vi "nanocal -- nuclear schottky fit V7.vi"() -> ()   [LabVIEW 2021] (continued)
\"B\" -> 0.000000000000   ,  \"θ\" -> 0.000000000000   ,  \"Reoff\" -> -959183.673469387924   ,  \"Imoff\" -> 0.000000000000   ,  \"στ1\" -> 0.000056019641   ,  \"στS\" -> 0.002791706038   ,  \"στN\" -> 0.000000650322    |>   , \r\"IDS0417_220525_RAW_cal__sam_\" ->   <|    \"ζ\" -> 0.020422056832   ,  \"τ1\" -> 0.006457484957   ,  \"τS\" -> 0.019722165301   ,  \"τN\" -> 0.000729413719   ,  \"τC\" -> 0.001622930071   ,  \"κ0\" -> 0.000000005380   ,  \"mm1\" -> 0.000030097695   ,  \"mm2\" -> 0.006162713408   ,  \"mm3\" -> 0.022756846254   ,  \"T\" -> 0.830000000000   ,  \"B\" -> 0.000000000000   ,  \"θ\" -> 0.000000000000   ,  \"Reoff\" -> -2081632.653061224150   ,  \"Imoff\" -> 0.000000000000   ,  \"στ1\" -> 0.000977899540   ,  \"στS\" -> 0.002370947727   ,  \"στN\" -> 0.000160479256    |>   , \r\"IDS0418_220525_RAW_cal__ref_\" ->   <|    \"ζ\" -> 0.101578237405   ,  \"τ1\" -> 0.000131000000   ,  \"τS\" -> 0.019496503151   ,  \"τN\" -> 0.000001000000   ,  \"τC\" -> 0.002824938622   ,  \"κ0\" -> 0.000000006490   ,  \"mm1\" -> 0.000130992305   ,  \"mm2\" -> 0.000232437503   ,  \"mm3\" -> 0.024070533970   ,  \"T\" -> 1.120000000000   ,  \"B\" -> 0.000000000000   ,  \"θ\" -> 0.000000000000   ,  \"Reoff\" -> -9469387.755102038390   ,  \"Imoff\" -> 0.000000000000   ,  \"στ1\" -> 0.000013096925   ,  \"στS\" -> 0.001629413974   ,  \"στN\" -> 0.000000279483    |>   , \r\"IDS0418_220525_RAW_cal__sam_\" ->   <|    \"ζ\" -> 0.010833914814   ,  \"τ1\" -> 0.006105280968   ,  \"τS\" -> 0.027771405990   ,  \"τN\" -> 0.000655710517   ,  \"τC\" -> 0.001898693697   ,  \"κ0\" -> 0.000000007420   ,  \"mm1\" -> 0.000019072683   ,  \"mm2\" -> 0.005941306089   ,  \"mm3\" -> 0.030778689359   ,  \"T\" -> 1.120000000000   ,  \"B\" -> 0.000000000000   ,  \"θ\" -> 0.000000000000   ,  \"Reoff\" -> -608163.265306122367   ,  \"Imoff\" -> 0.000000000000   ,  \"στ1\" -> 0.001326459237   ,  \"στS\" -> 0.003728359065   ,  \"στN\" -> 0.000181682896    |>   , \r\"IDS0419_220525_RAW_cal__ref_\" ->   <|    \"ζ\" -> 0.054328127598   ,  \"τ1\" -> 0.000131000000   ,  \"τS\" -> 0.041800630964   ,  \"τN\" -> 0.000001000000   ,  \"τC\" -> 0.008136787294   ,  \"κ0\" -> 0.000000011908   ,  \"mm1\" -> 0.000130996584   ,  \"mm2\" -> 0.000356366999   ,  \"mm3\" -> 0.051853059016   ,  \"T\" -> 1.900000000000   ,  \"B\" -> 0.000000000000   ,  \"θ\" -> 0.000000000000   ,  \"Reoff\" -> -2412244.897959183900   ,  \"Imoff\" -> 0.000000000000   ,  \"στ1\" -> 0.000075606348   ,  \"στS\" -> 0.006052354245   ,  \"στN\" -> 0.000000670558    |>   , \r\"IDS0419_220525_RAW_cal__sam_\" ->   <|    \"ζ\" -> 0.011595776290   ,  \"τ1\" -> 0.006117918264   ,  \"τS\" -> 0.061916055974   ,  \"τN\" -> 0.000669101537   ,  \"τC\" -> 0.002022450323   ,  \"κ0\" -> 0.000000012950   ,  \"mm1\" -> 0.000022465670   ,  \"mm2\" -> 0.006048051710   ,  \"mm3\" -> 0.065380732203   ,  \"T\" -> 1.900000000000   ,  \"B\" -> 0.000000000000   ,  \"θ\" -> 0.000000000000   ,  \"Reoff\" -> -608163.265306122367   ,  \"Imoff\" -> 0.000000000000   ,  \"στ1\" -> 0.001547930555   ,  \"στS\" -> 0.007827805463   ,  \"στN\" -> 0.000227173092    |>   , \r\"IDS0420_220525_RAW_cal__ref_\" ->   <|    \"ζ\" -> 0.054690281764   ,  \"τ1\" -> 0.000131000000   ,  \"τS\" -> 0.045992171451   ,  \"τN\" -> 0.000001000000   ,  \"τC\" -> 0.007372108350   ,  \"κ0\" -> 0.000000013567   ,  \"mm1\" -> 0.000130996911   ,  \"mm2\" -> 0.000333838788   ,  \"mm3\" -> 0.055546823607   ,  \"T\" -> 2.100000000000   ,  \"B\" -> 0.000000000000   ,  \"θ\" -> 0.000000000000   ,  \"Reoff\" -> -2412244.897959183900   ,  \"Imoff\" -> 0.000000000000   ,  \"στ1\" -> 0.000040532955   ,  \"στS\" -> 0.006090399823   ,  \"στN\" -> 0.000000564115    |>   , \r\"IDS0420_220525_RAW_cal__sam_\" ->   <|    \"ζ\" -> 0.011850996022   ,  \"τ1\" -> 0.005764384736   ,  \"τS\" -> 0.066220067505   ,  \"τN\" -> 0.000645440877   ,  \"τC\" -> 0.002901198812   ,  \"κ0\" -> 0.000000014700   ,  \"mm1\" -> 0.000032584327   ,  \"mm2\" -> 0.005706320364   ,  \"mm3\" -> 0.070584610113   ,  \"T\" -> 2.100000000000   ,  \"B\" -> 0.000000000000   ,  \"θ\" -> 0.000000000000   ,  \"Reoff\" -> -461224.489795918343   ,  \"Imoff\" -> 0.000000000000   ,  \"στ1\" -> 0.000879947943   ,  \"στS\" -> 0.005816006372   ,  \"στN\" -> 0.000150645668    |>   , \r\"IDS0421_220525_RAW_cal__ref_\" ->   <|    \"ζ\" -> 0.060508336123   ,  \"τ1\" -> 0.000131000000   ,  \"τS\" -> 0.007131357442   ,  \"τN\" -> 0.000001000000   ,  \"τC\" -> 0.009850008228   ,  \"κ0\" -> 0.000000015720   ,  \"mm1\" -> 0.000130969869   ,  \"mm2\" -> 0.000247654950   ,  \"mm3\" -> 0.017166307932   ,  \"T\" -> 2.300000000000   ,  \"B\" -> 0.000000000000   ,  \"θ\" -> 0.000000000000   ,  \"Reoff\" -> -391836.734693877398   ,  \"Imoff\" -> 0.000000000000   ,  \"στ1\" -> 0.000074085946   ,  \"στS\" -> 0.002081131924   ,  \"στN\" -> 0.000000819648    |>   , \r\"IDS0421_220525_RAW_cal__sam_\" ->   <|    \"ζ\" -> 0.017472306497   ,  \"τ1\" -> 0.005884707777   ,  \"τS\" -> 0.018273540555   ,  \"τN\" -> 0.000393530305   ,  \"τC\" -> 0.002873982576   ,  \"κ0\" -> 0.000000016000   ,  \"mm1\" -> 0.000042829990   ,  \"mm2\" -> 0.005738391469   ,  \"mm3\" -> 0.021970696537   ,  \"T\" -> 2.300000000000   ,  \"B\" -> 0.000000000000   ,  \"θ\" -> 0.000000000000   ,  \"Reoff\" -> -616326.530612244968   ,  \"Imoff\" -> 0.000000000000   ,  \"στ1\" -> 0.001449504442   ,  \"στS\" -> 0.003094967894   ,  \"στN\" -> 0.000132016087    |>   , \r\"IDS0422_220525_RAW_cal__ref_\" ->   <|    \"ζ\" -> 0.065958272689   ,  \"τ1\" -> 0.000131000000   ,  \"τS\" -> 0.004874385482   ,  \"τN\" -> 0.000001000000   ,  \"τC\" -> 0.006474262429   ,  \"κ0\" -> 0.000000022464   ,  \"mm1\" -> 0.000130934041   ,  \"mm2\" -> 0.000181249477   ,  \"mm3\" -> 0.011490036398   ,  \"T\" -> 3.100000000000   ,  \"B\" -> 0.000000000000   ,  \"θ\" -> 0.000000000000   ,  \"Reoff\" -> -391836.734693877398   ,  \"Imoff\" -> 0.000000000000   ,  \"στ1\" -> 0.000042174931   ,  \"στS\" -> 0.000833454188   ,  \"στN\" -> 0.000000451005    |>   , \r\"IDS0422_220525_RAW_cal__sam_\" ->   <|    \"ζ\" -> 0.013782660001   ,  \"τ1\" -> 0.005602489845   ,  \"τS\" -> 0.011122141420   ,  \"τN\" -> 0.000341635093   ,  \"τC\" -> 0.002887063483   ,  \"κ0\" -> 0.000000023500   ,  \"mm1\" -> 0.000031317292   ,  \"mm2\" -> 0.005389288482   ,  \"mm3\" -> 0.014690725401   ,  \"T\" -> 3.100000000000   ,  \"B\" -> 0.000000000000   ,  \"θ\" -> 0.000000000000   ,  \"Reoff\" -> -338775.510204081656   ,  \"Imoff\" -> 0.000000000000   ,  \"στ1\" -> 0.000787586702   ,  \"στS\" -> 0.001319427978   ,  \"στN\" -> 0.000072408344    |>   , \r\"IDS0424_220526_RAW_cal__ref_\" ->   <|    \"ζ\" -> 0.257865003377   ,  \"τ1\" -> 0.052975439100   ,  \"τS\" -> 0.072879585760   ,  \"τN\" -> 0.046129702285   ,  \"τC\" -> 0.000850997737   ,  \"κ0\" -> 0.000000000770   ,  \"mm1\" -> 0.000173173247   ,  \"mm2\" -> 0.027881728109   ,  \"mm3\" -> 0.175469153990   ,  \"T\" -> 0.190000000000   ,  \"B\" -> 10.000000000000   ,  \"θ\" -> 0.000000000000   ,  \"Reoff\" -> -49000000.000000000000   ,  \"Imoff\" -> 0.000000000000   ,  \"στ1\" -> 0.038419382366   ,  \"στS\" -> 0.010252018344   ,  \"στN\" -> 0.015460977129    |>   , \r\"IDS0424_220526_RAW_cal__sam_\" ->   <|    \"ζ\" -> 0.143096873941   ,  \"τ1\" -> 0.119527741552   ,  \"τS\" -> 0.213771204505   ,  \"τN\" -> 0.133065206622   ,  \"τC\" -> 0.001041786526   ,  \"κ0\" -> 0.000000000890   ,  \"mm1\" -> 0.000129929317   ,  \"mm2\" -> 0.064852834373   ,  \"mm3\" -> 0.452054381716   ,  \"T\" -> 0.190000000000   ,  \"B\" -> 10.000000000000   ,  \"θ\" -> 0.000000000000   ,  \"Reoff\" -> -41461224.489795915800   ,  \"Imoff\" -> 0.000000000000   ,  \"στ1\" -> 0.142328196867   ,  \"στS\" -> 0.153709890516   ,  \"στN\" -> 0.034979737706    |>   , \r\"IDS0425_220526_RAW_cal__ref_\" ->   <|    \"ζ\" -> 0.150640974704   ,  \"τ1\" -> 0.034197272609   ,  \"τS\" -> 0.049670713863   ,  \"τN\" -> 0.019296596370   ,  \"τC\" -> 0.000986151726   ,  \"κ0\" -> 0.000000001118   ,  \"mm1\" -> 0.000127191823   ,  \"mm2\" -> 0.021308290346   ,  \"mm3\" -> 0.093104555235   ,  \"T\" -> 0.250000000000   ,  \"B\" -> 10.000000000000   ,  \"θ\" -> 0.000000000000   ,  \"Reoff\" -> -20330612.244897961600   ,  \"Imoff\" -> 0.000000000000   ,  \"στ1\" -> 0.016426599332   ,  \"στS\" -> 0.002938321228   ,  \"στN\" -> 0.003825151273    |>   , \r\"IDS0425_220526_RAW_cal__sam_\" ->   <|    \"ζ\" -> 0.080613368975   ,  \"τ1\" -> 0.039981630615   ,  \"τS\" -> 0.067451052819   ,  \"τN\" -> 0.024952731947   ,  \"τC\" -> 0.001301901326   ,  \"κ0\" -> 0.000000001270   ,  \"mm1\" -> 0.000095538727   ,  \"mm2\" -> 0.025680137218   ,  \"mm3\" -> 0.115360621158   ,  \"T\" -> 0.250000000000   ,  \"B\" -> 10.000000000000   ,  \"θ\" -> 0.000000000000   ,  \"Reoff\" -> -15077551.020408168400   ,  \"Imoff\" -> 0.000000000000   ,  \"στ1\" -> 0.017921325903   ,  \"στS\" -> 0.008554959302   ,  \"στN\" -> 0.012696106226    |>   , \r\"IDS0426_220526_RAW_cal__ref_\" ->   <|    \"ζ\" -> 0.110651122840   ,  \"τ1\" -> 0.023688979566   ,  \"τS\" -> 0.041888104291   ,  \"τN\" -> 0.009400965947   ,  \"τC\" -> 0.001054144270   ,  \"κ0\" -> 0.000000001430   ,  \"mm1\" -> 0.000102915193   ,  \"mm2\" -> 0.017560405745   ,  \"mm3\" -> 0.064044066348   ,  \"T\" -> 0.300000000000   ,  \"B\" -> 10.000000000000   ,  \"θ\" -> 0.000000000000   ,  \"Reoff\" -> -13408163.265306122600   ,  \"Imoff\" -> 0.000000000000   ,  \"στ1\" -> 0.009988334429   ,  \"στS\" -> 0.001537868285   ,  \"στN\" -> 0.001719296338    |>   , \r\"IDS0426_220526_RAW_cal__sam_\" ->   <|    \"ζ\" -> 0.000000000000   ,  \"τ1\" -> 0.000000000000   ,  \"τS\" -> 0.000000000000   ,  \"τN\" -> 0.000000000000   ,  \"τC\" -> 0.000000000000   ,  \"κ0\" -> 0.000000000000   ,  \"mm1\" -> 0.000000000000   ,  \"mm2\" -> 0.000000000000   ,  \"mm3\" -> 0.000000000000   ,  \"T\" -> 0.300000000000   ,  \"B\" -> 10.000000000000   ,  \"θ\" -> 0.000000000000   ,  \"Reoff\" -> 0.000000000000   ,  \"Imoff\" -> 0.000000000000   ,  \"στ1\" -> 0.000000000000   ,  \"στS\" -> 0.000000000000   ,  \"στN\" -> 0.000000000000    |>   , \r\"IDS0427_220526_RAW_cal__ref_\" ->   <|    \"ζ\" -> 0.400378368532   ,  \"τ1\" -> 0.070020543839   ,  \"τS\" -> 0.131128875469   ,  \"τN\" -> 0.110503953528   ,  \"τC\" -> 0.000929381263   ,  \"κ0\" -> 0.000000000547   ,  \"mm1\" -> 0.000264755544   ,  \"mm2\" -> 0.034447529222   ,  \"mm3\" -> 0.374615027191   ,  \"T\" -> 0.150000000000   ,  \"B\" -> 10.000000000000   ,  \"θ\" -> 0.000000000000   ,  \"Reoff\" -> -90065306.122448980800   ,  \"Imoff\" -> 0.000000000000   ,  \"στ1\" -> 0.115545840550   ,  \"στS\" -> 0.062145974598   ,  \"στN\" -> 0.087083233243    |>   , \r\"IDS0427_220526_RAW_cal__sam_\" ->   <|    \"ζ\" -> 0.000000000000   ,  \"τ1\" -> 0.000000000000   ,  \"τS\" -> 0.000000000000   ,  \"τN\" -> 0.000000000000   ,  \"τC\" -> 0.000000000000   ,  \"κ0\" -> 0.000000000000   ,  \"mm1\" -> 0.000000000000   ,  \"mm2\" -> 0.000000000000   ,  \"mm3\" -> 0.000000000000   ,  \"T\" -> 0.150000000000   ,  \"B\" -> 10.000000000000   ,  \"θ\" -> 0.000000000000   ,  \"Reoff\" -> 0.000000000000   ,  \"Imoff\" -> 0.000000000000   ,  \"στ1\" -> 0.000000000000   ,  \"στS\" -> 0.000000000000   ,  \"στN\" -> 0.000000000000    |>   , \r\"IDS0428_220526_RAW_cal__ref_\" ->   <|    \"ζ\" -> 0.082438962756   ,  \"τ1\" -> 0.024345135189   ,  \"τS\" -> 0.039010983719   ,  \"τN\" -> 0.005604008996   ,  \"τC\" -> 0.001011795266   ,  \"κ0\" -> 0.000000001850   ,  \"mm1\" -> 0.000075386231   ,  \"mm2\" -> 0.019395489677   ,  \"mm3\" -> 0.054179060985   ,  \"T\" -> 0.360000000000   ,  \"B\" -> 10.000000000000   ,  \"θ\" -> 0.000000000000   ,  \"Reoff\" -> -9632653.061224490410   ,  \"Imoff\" -> 0.000000000000   ,  \"στ1\" -> 0.001903743103   ,  \"στS\" -> 0.000574153374   ,  \"στN\" -> 0.002568840036    |>   , \r\"IDS0428_220526_RAW_cal__sam_\" ->   <|    \"ζ\" -> 0.000000000000   ,  \"τ1\" -> 0.000000000000   ,  \"τS\" -> 0.000000000000   ,  \"τN\" -> 0.000000000000   ,  \"τC\" -> 0.000000000000   ,  \"κ0\" -> 0.000000000000   ,  \"mm1\" -> 0.000000000000   ,  \"mm2\" -> 0.000000000000   ,  \"mm3\" -> 0.000000000000   ,  \"T\" -> 0.360000000000   ,  \"B\" -> 10.000000000000   ,  \"θ\" -> 0.000000000000   ,  \"Reoff\" -> 0.000000000000   ,  \"Imoff\" -> 0.000000000000   ,  \"στ1\" -> 0.000000000000   ,  \"στS\" -> 0.000000000000   ,  \"στN\" -> 0.000000000000    |>   , \r\"IDS0429_220526_RAW_cal__ref_\" ->   <|    \"ζ\" -> 0.070312011413   ,  \"τ1\" -> 0.022685637424   ,  \"τS\" -> 0.038017817435   ,  \"τN\" -> 0.003686111033   ,  \"τC\" -> 0.000858092615   ,  \"κ0\" -> 0.000000002230   ,  \"mm1\" -> 0.000055279779   ,  \"mm2\" -> 0.019266175315   ,  \"mm3\" -> 0.048858490507   ,  \"T\" -> 0.420000000000   ,  \"B\" -> 10.000000000000   ,  \"θ\" -> 0.000000000000   ,  \"Reoff\" -> -9632653.061224490410   ,  \"Imoff\" -> 0.000000000000   ,  \"στ1\" -> 0.001355990341   ,  \"στS\" -> 0.000271524957   ,  \"στN\" -> 0.000140246830    |>   , \r\"IDS0429_220526_RAW_cal__sam_\" ->   <|    \"ζ\" -> 0.000000000000   ,  \"τ1\" -> 0.000000000000   ,  \"τS\" -> 0.000000000000   ,  \"τN\" -> 0.000000000000   ,  \"τC\" -> 0.000000000000   ,  \"κ0\" -> 0.000000000000   ,  \"mm1\" -> 0.000000000000   ,  \"mm2\" -> 0.000000000000   ,  \"mm3\" -> 0.000000000000   ,  \"T\" -> 0.420000000000   ,  \"B\" -> 10.000000000000   ,  \"θ\" -> 0.000000000000   ,  \"Reoff\" -> 0.000000000000   ,  \"Imoff\" -> 0.000000000000   ,  \"στ1\" -> 0.000000000000   ,  \"στS\" -> 0.000000000000   ,  \"στN\" -> 0.000000000000    |>   , \r\"IDS0430_220526_RAW_cal__ref_\" ->   <|    \"ζ\" -> 0.045461152604   ,  \"τ1\" -> 0.022205538452   ,  \"τS\" -> 0.038393095410   ,  \"τN\" -> 0.002129809404   ,  \"τC\" -> 0.001500655488   ,  \"κ0\" -> 0.000000002910   ,  \"mm1\" -> 0.000062998174   ,  \"mm2\" -> 0.020118168551   ,  \"mm3\" -> 0.045890149989   ,  \"T\" -> 0.520000000000   ,  \"B\" -> 10.000000000000   ,  \"θ\" -> 0.000000000000   ,  \"Reoff\" -> -3224489.795918375260   ,  \"Imoff\" -> 0.000000000000   ,  \"στ1\" -> 0.001544196925   ,  \"στS\" -> 0.000197668706   ,  \"στN\" -> 0.000070756968    |>   , \r\"IDS0430_220526_RAW_cal__sam_\" ->   <|    \"ζ\" -> 0.000000000000   ,  \"τ1\" -> 0.000000000000   ,  \"τS\" -> 0.000000000000   ,  \"τN\" -> 0.000000000000   ,  \"τC\" -> 0.000000000000   ,  \"κ0\" -> 0.000000000000   ,  \"mm1\" -> 0.000000000000   ,  \"mm2\" -> 0.000000000000   ,  \"mm3\" -> 0.000000000000   ,  \"T\" -> 0.520000000000   ,  \"B\" -> 10.000000000000   ,  \"θ\" -> 0.000000000000   ,  \"Reoff\" -> 0.000000000000   ,  \"Imoff\" -> 0.000000000000   ,  \"στ1\" -> 0.000000000000   ,  \"στS\" -> 0.000000000000   ,  \"στN\" -> 0.000000000000    |>   , \r\"IDS0431_220527_RAW_cal__ref_\" ->   <|    \"ζ\" -> 0.560959524386   ,  \"τ1\" -> 0.162135875123   ,  \"τS\" -> 0.311559023690   ,  \"τN\" -> 0.235565493895   ,  \"τC\" -> 0.000943331482   ,  \"κ0\" -> 0.000000000415   ,  \"mm1\" -> 0.000338581832   ,  \"mm2\" -> 0.084703245290   ,  \"mm3\" -> 0.932076606233   ,  \"T\" -> 0.120000000000   ,  \"B\" -> 10.000000000000   ,  \"θ\" -> 0.000000000000   ,  \"Reoff\" -> -130387755.102040812000   ,  \"Imoff\" -> 0.000000000000   ,  \"στ1\" -> 0.196821258023   ,  \"στS\" -> 0.124985342591   ,  \"στN\" -> 0.122755892139    |>   , \r\"IDS0431_220527_RAW_cal__sam_\" ->   <|    \"ζ\" -> 0.000000000000   ,  \"τ1\" -> 0.000000000000   ,  \"τS\" -> 0.000000000000   ,  \"τN\" -> 0.000000000000   ,  \"τC\" -> 0.000000000000   ,  \"κ0\" -> 0.000000000000   ,  \"mm1\" -> 0.000000000000   ,  \"mm2\" -> 0.000000000000   ,  \"mm3\" -> 0.000000000000   ,  \"T\" -> 0.120000000000   ,  \"B\" -> 10.000000000000   ,  \"θ\" -> 0.000000000000   ,  \"Reoff\" -> 0.000000000000   ,  \"Imoff\" -> 0.000000000000   ,  \"στ1\" -> 0.000000000000   ,  \"στS\" -> 0.000000000000   ,  \"στN\" -> 0.000000000000    |>   , \r\"IDS0432_220527_RAW_cal__ref_\" ->   <|    \"ζ\" -> 0.302881771202   ,  \"τ1\" -> 0.053970650610   ,  \"τS\" -> 0.084832458604   ,  \"τN\" -> 0.070036651320   ,  \"τC\" -> 0.000864371133   ,  \"κ0\" -> 0.000000000675   ,  \"mm1\" -> 0.000199736141   ,  \"mm2\" -> 0.026051282095   ,  \"mm3\" -> 0.230360143749   ,  \"T\" -> 0.170000000000   ,  \"B\" -> 10.000000000000   ,  \"θ\" -> 0.000000000000   ,  \"Reoff\" -> -65714285.714285716400   ,  \"Imoff\" -> 0.000000000000   ,  \"στ1\" -> 0.042116863127   ,  \"στS\" -> 0.016985307293   ,  \"στN\" -> 0.023565277591    |>   , \r\"IDS0432_220527_RAW_cal__sam_\" ->   <|    \"ζ\" -> 0.000000000000   ,  \"τ1\" -> 0.000000000000   ,  \"τS\" -> 0.000000000000   ,  \"τN\" -> 0.000000000000   ,  \"τC\" -> 0.000000000000   ,  \"κ0\" -> 0.000000000000   ,  \"mm1\" -> 0.000000000000   ,  \"mm2\" -> 0.000000000000   ,  \"mm3\" -> 0.000000000000   ,  \"T\" -> 0.170000000000   ,  \"B\" -> 10.000000000000   ,  \"θ\" -> 0.000000000000   ,  \"Reoff\" -> 0.000000000000   ,  \"Imoff\" -> 0.000000000000   ,  \"στ1\" -> 0.000000000000   ,  \"στS\" -> 0.000000000000   ,  \"στN\" -> 0.000000000000    |>   , \r\"IDS0433_220527_RAW_cal__ref_\" ->   <|    \"ζ\" -> 0.035999178559   ,  \"τ1\" -> 0.021236822586   ,  \"τS\" -> 0.040779763241   ,  \"τN\" -> 0.001074221992   ,  \"τC\" -> 0.001739718615   ,  \"κ0\" -> 0.000000003576   ,  \"mm1\" -> 0.000058137989   ,  \"mm2\" -> 0.020282386509   ,  \"mm3\" -> 0.045996711024   ,  \"T\" -> 0.620000000000   ,  \"B\" -> 10.000000000000   ,  \"θ\" -> 0.000000000000   ,  \"Reoff\" -> -1959183.673469394450   ,  \"Imoff\" -> 0.000000000000   ,  \"στ1\" -> 0.001449693425   ,  \"στS\" -> 0.000173563135   ,  \"στN\" -> 0.000045450535    |>   , \r\"IDS0433_220527_RAW_cal__sam_\" ->   <|    \"ζ\" -> 0.000000000000   ,  \"τ1\" -> 0.000000000000   ,  \"τS\" -> 0.000000000000   ,  \"τN\" -> 0.000000000000   ,  \"τC\" -> 0.000000000000   ,  \"κ0\" -> 0.000000000000   ,  \"mm1\" -> 0.000000000000   ,  \"mm2\" -> 0.000000000000   ,  \"mm3\" -> 0.000000000000   ,  \"T\" -> 0.620000000000   ,  \"B\" -> 10.000000000000   ,  \"θ\" -> 0.000000000000   ,  \"Reoff\" -> 0.000000000000   ,  \"Imoff\" -> 0.000000000000   ,  \"στ1\" -> 0.000000000000   ,  \"στS\" -> 0.000000000000   ,  \"στN\" -> 0.000000000000    |>   , \r\"IDS0434_220527_RAW_cal__ref_\" ->   <|    \"ζ\" -> 0.027519355554   ,  \"τ1\" -> 0.020590521074   ,  \"τS\" -> 0.048137141101   ,  \"τN\" -> 0.000693113139   ,  \"τC\" -> 0.001789335146   ,  \"κ0\" -> 0.000000004950   ,  \"mm1\" -> 0.000046291190   ,  \"mm2\" -> 0.020129239579   ,  \"mm3\" -> 0.052378356819   ,  \"T\" -> 0.820000000000   ,  \"B\" -> 10.000000000000   ,  \"θ\" -> 0.000000000000   ,  \"Reoff\" -> -1326530.612244904040   ,  \"Imoff\" -> 0.000000000000   ,  \"στ1\" -> 0.000620759114   ,  \"στS\" -> 0.000219619310   ,  \"στN\" -> 0.000010903062    |>   , \r\"IDS0434_220527_RAW_cal__sam_\" ->   <|    \"ζ\" -> 0.000000000000   ,  \"τ1\" -> 0.000000000000   ,  \"τS\" -> 0.000000000000   ,  \"τN\" -> 0.000000000000   ,  \"τC\" -> 0.000000000000   ,  \"κ0\" -> 0.000000000000   ,  \"mm1\" -> 0.000000000000   ,  \"mm2\" -> 0.000000000000   ,  \"mm3\" -> 0.000000000000   ,  \"T\" -> 0.820000000000   ,  \"B\" -> 10.000000000000   ,  \"θ\" -> 0.000000000000   ,  \"Reoff\" -> 0.000000000000   ,  \"Imoff\" -> 0.000000000000   ,  \"στ1\" -> 0.000000000000   ,  \"στS\" -> 0.000000000000   ,  \"στN\" -> 0.000000000000    |>   , \r\"IDS0435_220527_RAW_cal__ref_\" ->   <|    \"ζ\" -> 0.020842861739   ,  \"τ1\" -> 0.020135384195   ,  \"τS\" -> 0.018612634604   ,  \"τN\" -> 0.000305402785   ,  \"τC\" -> 0.002204389625   ,  \"κ0\" -> 0.000000007040   ,  \"mm1\" -> 0.000040405722   ,  \"mm2\" -> 0.018212466466   ,  \"mm3\" -> 0.023399245059   ,  \"T\" -> 1.120000000000   ,  \"B\" -> 10.000000000000   ,  \"θ\" -> 0.000000000000   ,  \"Reoff\" -> -693877.551020413636   ,  \"Imoff\" -> 0.000000000000   ,  \"στ1\" -> 0.001444867016   ,  \"στS\" -> 0.000117188914   ,  \"στN\" -> 0.000006503631    |>   , \r\"IDS0435_220527_RAW_cal__sam_\" ->   <|    \"ζ\" -> 0.000000000000   ,  \"τ1\" -> 0.000000000000   ,  \"τS\" -> 0.000000000000   ,  \"τN\" -> 0.000000000000   ,  \"τC\" -> 0.000000000000   ,  \"κ0\" -> 0.000000000000   ,  \"mm1\" -> 0.000000000000   ,  \"mm2\" -> 0.000000000000   ,  \"mm3\" -> 0.000000000000   ,  \"T\" -> 1.120000000000   ,  \"B\" -> 10.000000000000   ,  \"θ\" -> 0.000000000000   ,  \"Reoff\" -> 0.000000000000   ,  \"Imoff\" -> 0.000000000000   ,  \"στ1\" -> 0.000000000000   ,  \"στS\" -> 0.000000000000   ,  \"στN\" -> 0.000000000000    |>   , \r\"IDS0436_220527_RAW_cal__ref_\" ->   <|    \"ζ\" -> 0.020634042480   ,  \"τ1\" -> 0.020416898580   ,  \"τS\" -> 0.013006754143   ,  \"τN\" -> 0.000157221748   ,  \"τC\" -> 0.001868338850   ,  \"κ0\" -> 0.000000012250   ,  \"mm1\" -> 0.000033184482   ,  \"mm2\" -> 0.014698009084   ,  \"mm3\" -> 0.020989645793   ,  \"T\" -> 1.900000000000   ,  \"B\" -> 10.000000000000   ,  \"θ\" -> 0.000000000000   ,  \"Reoff\" -> -693877.551020413636   ,  \"Imoff\" -> 0.000000000000   ,  \"στ1\" -> 0.001009802597   ,  \"στS\" -> 0.000108538250   ,  \"στN\" -> 0.000005592624    |>   , \r\"IDS0436_220527_RAW_cal__sam_\" ->   <|    \"ζ\" -> 0.000000000000   ,  \"τ1\" -> 0.000000000000   ,  \"τS\" -> 0.000000000000   ,  \"τN\" -> 0.000000000000   ,  \"τC\" -> 0.000000000000   ,  \"κ0\" -> 0.000000000000   ,  \"mm1\" -> 0.000000000000   ,  \"mm2\" -> 0.000000000000   ,  \"mm3\" -> 0.000000000000   ,  \"T\" -> 1.900000000000   ,  \"B\" -> 10.000000000000   ,  \"θ\" -> 0.000000000000   ,  \"Reoff\" -> 0.000000000000   ,  \"Imoff\" -> 0.000000000000   ,  \"στ1\" -> 0.000000000000   ,  \"στS\" -> 0.000000000000   ,  \"στN\" -> 0.000000000000    |>   , \r\"IDS0437_220527_RAW_cal__ref_\" ->   <|    \"ζ\" -> 0.017700486500   ,  \"τ1\" -> 0.021195716861   ,  \"τS\" -> 0.009553240691   ,  \"τN\" -> 0.000096318625   ,  \"τC\" -> 0.001777778444   ,  \"κ0\" -> 0.000000022000   ,  \"mm1\" -> 0.000026199986   ,  \"mm2\" -> 0.011360732885   ,  \"mm3\" -> 0.021406923644   ,  \"T\" -> 3.100000000000   ,  \"B\" -> 10.000000000000   ,  \"θ\" -> 0.000000000000   ,  \"Reoff\" -> -326530.612244898453   ,  \"Imoff\" -> 0.000000000000   ,  \"στ1\" -> 0.003823035587   ,  \"στS\" -> 0.000080670014   ,  \"στN\" -> 0.000008312416    |>   , \r\"IDS0437_220527_RAW_cal__sam_\" ->   <|    \"ζ\" -> 0.000000000000   ,  \"τ1\" -> 0.000000000000   ,  \"τS\" -> 0.000000000000   ,  \"τN\" -> 0.000000000000   ,  \"τC\" -> 0.000000000000   ,  \"κ0\" -> 0.000000000000   ,  \"mm1\" -> 0.000000000000   ,  \"mm2\" -> 0.000000000000   ,  \"mm3\" -> 0.000000000000   ,  \"T\" -> 3.100000000000   ,  \"B\" -> 10.000000000000   ,  \"θ\" -> 0.000000000000   ,  \"Reoff\" -> 0.000000000000   ,  \"Imoff\" -> 0.000000000000   ,  \"στ1\" -> 0.000000000000   ,  \"στS\" -> 0.000000000000   ,  \"στN\" -> 0.000000000000    |>   , \r\"IDS0438_220527_RAW_cal__ref_\" ->   <|    \"ζ\" -> 0.017333863476   ,  \"τ1\" -> 0.021487771905   ,  \"τS\" -> 0.006060943357   ,  \"τN\" -> 0.000094743973   ,  \"τC\" -> 0.001680463551   ,  \"κ0\" -> 0.000000054800   ,  \"mm1\" -> 0.000022565233   ,  \"mm2\" -> 0.007769356044   ,  \"mm3\" -> 0.021638703353   ,  \"T\" -> 5.700000000000   ,  \"B\" -> 10.000000000000   ,  \"θ\" -> 0.000000000000   ,  \"Reoff\" -> -102040.816326530650   ,  \"Imoff\" -> 0.000000000000   ,  \"στ1\" -> 0.003634760564   ,  \"στS\" -> 0.000066823566   ,  \"στN\" -> 0.000004946508    |>   , \r\"IDS0438_220527_RAW_cal__sam_\" ->   <|    \"ζ\" -> 0.000000000000   ,  \"τ1\" -> 0.000000000000   ,  \"τS\" -> 0.000000000000   ,  \"τN\" -> 0.000000000000   ,  \"τC\" -> 0.000000000000   ,  \"κ0\" -> 0.000000000000   ,  \"mm1\" -> 0.000000000000   ,  \"mm2\" -> 0.000000000000   ,  \"mm3\" -> 0.000000000000   ,  \"T\" -> 5.700000000000   ,  \"B\" -> 10.000000000000   ,  \"θ\" -> 0.000000000000   ,  \"Reoff\" -> 0.000000000000   ,  \"Imoff\" -> 0.000000000000   ,  \"στ1\" -> 0.000000000000   ,  \"στS\" -> 0.000000000000   ,  \"στN\" -> 0.000000000000    |>   , \r\"IDS0439_220527_RAW_cal__ref_\" ->   <|    \"ζ\" -> 0.020515660719   ,  \"τ1\" -> 0.020182411708   ,  \"τS\" -> 0.016419895032   ,  \"τN\" -> 0.000240616919   ,  \"τC\" -> 0.002259910162   ,  \"κ0\" -> 0.000000008010   ,  \"mm1\" -> 0.000040116981   ,  \"mm2\" -> 0.017425178232   ,  \"mm3\" -> 0.021979340018   ,  \"T\" -> 1.280000000000   ,  \"B\" -> 10.000000000000   ,  \"θ\" -> 0.000000000000   ,  \"Reoff\" -> -693877.551020413636   ,  \"Imoff\" -> 0.000000000000   ,  \"στ1\" -> 0.001720696083   ,  \"στS\" -> 0.000105898596   ,  \"στN\" -> 0.000011441558    |>   , \r\"IDS0439_220527_RAW_cal__sam_\" ->   <|    \"ζ\" -> 0.000000000000   ,  \"τ1\" -> 0.000000000000   ,  \"τS\" -> 0.000000000000   ,  \"τN\" -> 0.000000000000   ,  \"τC\" -> 0.000000000000   ,  \"κ0\" -> 0.000000000000   ,  \"mm1\" -> 0.000000000000   ,  \"mm2\" -> 0.000000000000   ,  \"mm3\" -> 0.000000000000   ,  \"T\" -> 1.280000000000   ,  \"B\" -> 10.000000000000   ,  \"θ\" -> 0.000000000000   ,  \"Reoff\" -> 0.000000000000   ,  \"Imoff\" -> 0.000000000000   ,  \"στ1\" -> 0.000000000000   ,  \"στS\" -> 0.000000000000   ,  \"στN\" -> 0.000000000000    |>   , \r\"IDS0441_220527_RAW_cal__ref_\" ->   <|    \"ζ\" -> 0.211856799532   ,  \"τ1\" -> 0.173713031248   ,  \"τS\" -> 0.025047077219   ,  \"τN\" -> 0.022799850294   ,  \"τC\" -> 0.001119487792   ,  \"κ0\" -> 0.000000000820   ,  \"mm1\" -> 0.000189887587   ,  \"mm2\" -> 0.026344768969   ,  \"mm3\" -> 0.206281486927   ,  \"T\" -> 0.200000000000   ,  \"B\" -> 6.000000000000   ,  \"θ\" -> 0.000000000000   ,  \"Reoff\" -> -7510204.081632658840   ,  \"Imoff\" -> 0.000000000000   ,  \"στ1\" -> 0.033514341427   ,  \"στS\" -> 0.000356628888   ,  \"στN\" -> 0.003953255270    |>   , \r\"IDS0441_220527_RAW_cal__sam_\" ->   <|    \"ζ\" -> 0.000000000000   ,  \"τ1\" -> 0.000000000000   ,  \"τS\" -> 0.000000000000   ,  \"τN\" -> 0.000000000000   ,  \"τC\" -> 0.000000000000   ,  \"κ0\" -> 0.000000000000   ,  \"mm1\" -> 0.000000000000   ,  \"mm2\" -> 0.000000000000   ,  \"mm3\" -> 0.000000000000   ,  \"T\" -> 0.200000000000   ,  \"B\" -> 6.000000000000   ,  \"θ\" -> 0.000000000000   ,  \"Reoff\" -> 0.000000000000   ,  \"Imoff\" -> 0.000000000000   ,  \"στ1\" -> 0.000000000000   ,  \"στS\" -> 0.000000000000   ,  \"στN\" -> 0.000000000000    |>   , \r\"IDS0442_220528_RAW_cal__ref_\" ->   <|    \"ζ\" -> 0.627289985820   ,  \"τ1\" -> 0.239743496780   ,  \"τS\" -> 0.076926495749   ,  \"τN\" -> 0.159415903746   ,  \"τC\" -> 0.000763641667   ,  \"κ0\" -> 0.000000000435   ,  \"mm1\" -> 0.000293264880   ,  \"mm2\" -> 0.052650493650   ,  \"mm3\" -> 0.572160999840   ,  \"T\" -> 0.120000000000   ,  \"B\" -> 6.000000000000   ,  \"θ\" -> 0.000000000000   ,  \"Reoff\" -> -187755102.040816367000   ,  \"Imoff\" -> 0.000000000000   ,  \"στ1\" -> 0.245568364347   ,  \"στS\" -> 0.022170590915   ,  \"στN\" -> 0.126655465898    |>   , \r\"IDS0442_220528_RAW_cal__sam_\" ->   <|    \"ζ\" -> 0.000000000000   ,  \"τ1\" -> 0.000000000000   ,  \"τS\" -> 0.000000000000   ,  \"τN\" -> 0.000000000000   ,  \"τC\" -> 0.000000000000   ,  \"κ0\" -> 0.000000000000   ,  \"mm1\" -> 0.000000000000   ,  \"mm2\" -> 0.000000000000   ,  \"mm3\" -> 0.000000000000   ,  \"T\" -> 0.120000000000   ,  \"B\" -> 6.000000000000   ,  \"θ\" -> 0.000000000000   ,  \"Reoff\" -> 0.000000000000   ,  \"Imoff\" -> 0.000000000000   ,  \"στ1\" -> 0.000000000000   ,  \"στS\" -> 0.000000000000   ,  \"στN\" -> 0.000000000000    |>   , \r\"IDS0443_220528_RAW_cal__ref_\" ->   <|    \"ζ\" -> 0.436035823116   ,  \"τ1\" -> 0.136298324856   ,  \"τS\" -> 0.035428802447   ,  \"τN\" -> 0.042141009445   ,  \"τC\" -> 0.000863434496   ,  \"κ0\" -> 0.000000000631   ,  \"mm1\" -> 0.000259087412   ,  \"mm2\" -> 0.032519927017   ,  \"mm3\" -> 0.215775773592   ,  \"T\" -> 0.150000000000   ,  \"B\" -> 6.000000000000   ,  \"θ\" -> 0.000000000000   ,  \"Reoff\" -> -60040816.326530613000   ,  \"Imoff\" -> 0.000000000000   ,  \"στ1\" -> 0.080047050506   ,  \"στS\" -> 0.002312030387   ,  \"στN\" -> 0.019370507574    |>   , \r\"IDS0443_220528_RAW_cal__sam_\" ->   <|    \"ζ\" -> 0.000000000000   ,  \"τ1\" -> 0.000000000000   ,  \"τS\" -> 0.000000000000   ,  \"τN\" -> 0.000000000000   ,  \"τC\" -> 0.000000000000   ,  \"κ0\" -> 0.000000000000   ,  \"mm1\" -> 0.000000000000   ,  \"mm2\" -> 0.000000000000   ,  \"mm3\" -> 0.000000000000   ,  \"T\" -> 0.150000000000   ,  \"B\" -> 6.000000000000   ,  \"θ\" -> 0.000000000000   ,  \"Reoff\" -> 0.000000000000   ,  \"Imoff\" -> 0.000000000000   ,  \"στ1\" -> 0.000000000000   ,  \"στS\" -> 0.000000000000   ,  \"στN\" -> 0.000000000000    |>   , \r\"IDS0444_220528_RAW_cal__ref_\" ->   <|    \"ζ\" -> 0.312738827075   ,  \"τ1\" -> 0.153166775684   ,  \"τS\" -> 0.029428403772   ,  \"τN\" -> 0.032059842595   ,  \"τC\" -> 0.000966119229   ,  \"κ0\" -> 0.000000000763   ,  \"mm1\" -> 0.000225827852   ,  \"mm2\" -> 0.029383297615   ,  \"mm3\" -> 0.205241777861   ,  \"T\" -> 0.170000000000   ,  \"B\" -> 6.000000000000   ,  \"θ\" -> 0.000000000000   ,  \"Reoff\" -> -20979591.836734697200   ,  \"Imoff\" -> 0.000000000000   ,  \"στ1\" -> 0.194871487206   ,  \"στS\" -> 0.001481931895   ,  \"στN\" -> 0.032515587695    |>   , \r\"IDS0444_220528_RAW_cal__sam_\" ->   <|    \"ζ\" -> 0.000000000000   ,  \"τ1\" -> 0.000000000000   ,  \"τS\" -> 0.000000000000   ,  \"τN\" -> 0.000000000000   ,  \"τC\" -> 0.000000000000   ,  \"κ0\" -> 0.000000000000   ,  \"mm1\" -> 0.000000000000   ,  \"mm2\" -> 0.000000000000   ,  \"mm3\" -> 0.000000000000   ,  \"T\" -> 0.170000000000   ,  \"B\" -> 6.000000000000   ,  \"θ\" -> 0.000000000000   ,  \"Reoff\" -> 0.000000000000   ,  \"Imoff\" -> 0.000000000000   ,  \"στ1\" -> 0.000000000000   ,  \"στS\" -> 0.000000000000   ,  \"στN\" -> 0.000000000000    |>   , \r\"IDS0445_220528_RAW_cal__ref_\" ->   <|    \"ζ\" -> 0.144974292956   ,  \"τ1\" -> 0.278153679109   ,  \"τS\" -> 0.020087180736   ,  \"τN\" -> 0.018878235169   ,  \"τC\" -> 0.001360650262   ,  \"κ0\" -> 0.000000001251   ,  \"mm1\" -> 0.000163756081   ,  \"mm2\" -> 0.022311875645   ,  \"mm3\" -> 0.301653097172   ,  \"T\" -> 0.250000000000   ,  \"B\" -> 6.000000000000   ,  \"θ\" -> 0.000000000000   ,  \"Reoff\" -> -857142.857142856343   ,  \"Imoff\" -> 0.000000000000   ,  \"στ1\" -> 0.021844314170   ,  \"στS\" -> 0.000158941721   ,  \"στN\" -> 0.001374609128    |>   , \r\"IDS0445_220528_RAW_cal__sam_\" ->   <|    \"ζ\" -> 0.000000000000   ,  \"τ1\" -> 0.000000000000   ,  \"τS\" -> 0.000000000000   ,  \"τN\" -> 0.000000000000   ,  \"τC\" -> 0.000000000000   ,  \"κ0\" -> 0.000000000000   ,  \"mm1\" -> 0.000000000000   ,  \"mm2\" -> 0.000000000000   ,  \"mm3\" -> 0.000000000000   ,  \"T\" -> 0.250000000000   ,  \"B\" -> 6.000000000000   ,  \"θ\" -> 0.000000000000   ,  \"Reoff\" -> 0.000000000000   ,  \"Imoff\" -> 0.000000000000   ,  \"στ1\" -> 0.000000000000   ,  \"στS\" -> 0.000000000000   ,  \"στN\" -> 0.000000000000    |>   , \r\"IDS0446_220528_RAW_cal__ref_\" ->   <|    \"ζ\" -> 0.103205072553   ,  \"τ1\" -> 0.456877167810   ,  \"τS\" -> 0.018190810680   ,  \"τN\" -> 0.020353539569   ,  \"τC\" -> 0.001532633678   ,  \"κ0\" -> 0.000000001557   ,  \"mm1\" -> 0.000134033999   ,  \"mm2\" -> 0.020416907251   ,  \"mm3\" -> 0.480381182951   ,  \"T\" -> 0.300000000000   ,  \"B\" -> 6.000000000000   ,  \"θ\" -> 0.000000000000   ,  \"Reoff\" -> -461224.489795918343   ,  \"Imoff\" -> 0.000000000000   ,  \"στ1\" -> 0.032347659490   ,  \"στS\" -> 0.000102258041   ,  \"στN\" -> 0.001172701872    |>   , \r\"IDS0446_220528_RAW_cal__sam_\" ->   <|    \"ζ\" -> 0.000000000000   ,  \"τ1\" -> 0.000000000000   ,  \"τS\" -> 0.000000000000   ,  \"τN\" -> 0.000000000000   ,  \"τC\" -> 0.000000000000   ,  \"κ0\" -> 0.000000000000   ,  \"mm1\" -> 0.000000000000   ,  \"mm2\" -> 0.000000000000   ,  \"mm3\" -> 0.000000000000   ,  \"T\" -> 0.300000000000   ,  \"B\" -> 6.000000000000   ,  \"θ\" -> 0.000000000000   ,  \"Reoff\" -> 0.000000000000   ,  \"Imoff\" -> 0.000000000000   ,  \"στ1\" -> 0.000000000000   ,  \"στS\" -> 0.000000000000   ,  \"στN\" -> 0.000000000000    |>   , \r\"IDS0447_220528_RAW_cal__ref_\" ->   <|    \"ζ\" -> 0.067386498273   ,  \"τ1\" -> 0.033759383158   ,  \"τS\" -> 0.016352467508   ,  \"τN\" -> 0.000055602042   ,  \"τC\" -> 0.002052818742   ,  \"κ0\" -> 0.000000002053   ,  \"mm1\" -> 0.000116658355   ,  \"mm2\" -> 0.019311291178   ,  \"mm3\" -> 0.033898004267   ,  \"T\" -> 0.360000000000   ,  \"B\" -> 6.000000000000   ,  \"θ\" -> 0.000000000000   ,  \"Reoff\" -> 4122448.979591837150   ,  \"Imoff\" -> 0.000000000000   ,  \"στ1\" -> 0.002480419110   ,  \"στS\" -> 0.000128292028   ,  \"στN\" -> 0.000001339614    |>   , \r\"IDS0447_220528_RAW_cal__sam_\" ->   <|    \"ζ\" -> 0.000000000000   ,  \"τ1\" -> 0.000000000000   ,  \"τS\" -> 0.000000000000   ,  \"τN\" -> 0.000000000000   ,  \"τC\" -> 0.000000000000   ,  \"κ0\" -> 0.000000000000   ,  \"mm1\" -> 0.000000000000   ,  \"mm2\" -> 0.000000000000   ,  \"mm3\" -> 0.000000000000   ,  \"T\" -> 0.360000000000   ,  \"B\" -> 6.000000000000   ,  \"θ\" -> 0.000000000000   ,  \"Reoff\" -> 0.000000000000   ,  \"Imoff\" -> 0.000000000000   ,  \"στ1\" -> 0.000000000000   ,  \"στS\" -> 0.000000000000   ,  \"στN\" -> 0.000000000000    |>   , \r\"IDS0448_220528_RAW_cal__ref_\" ->   <|    \"ζ\" -> 0.022507492936   ,  \"τ1\" -> 0.033871434243   ,  \"τS\" -> 0.016835987173   ,  \"τN\" -> 0.000213468402   ,  \"τC\" -> 0.001778165835   ,  \"κ0\" -> 0.000000002480   ,  \"mm1\" -> 0.000035543102   ,  \"mm2\" -> 0.018688914469   ,  \"mm3\" -> 0.034358338584   ,  \"T\" -> 0.420000000000   ,  \"B\" -> 6.000000000000   ,  \"θ\" -> 0.000000000000   ,  \"Reoff\" -> 4122448.979591837150   ,  \"Imoff\" -> 0.000000000000   ,  \"στ1\" -> 0.007814821926   ,  \"στS\" -> 0.000385740474   ,  \"στN\" -> 0.000018309382    |>   , \r\"IDS0448_220528_RAW_cal__sam_\" ->   <|    \"ζ\" -> 0.000000000000   ,  \"τ1\" -> 0.000000000000   ,  \"τS\" -> 0.000000000000   ,  \"τN\" -> 0.000000000000   ,  \"τC\" -> 0.000000000000   ,  \"κ0\" -> 0.000000000000   ,  \"mm1\" -> 0.000000000000   ,  \"mm2\" -> 0.000000000000   ,  \"mm3\" -> 0.000000000000   ,  \"T\" -> 0.420000000000   ,  \"B\" -> 6.000000000000   ,  \"θ\" -> 0.000000000000   ,  \"Reoff\" -> 0.000000000000   ,  \"Imoff\" -> 0.000000000000   ,  \"στ1\" -> 0.000000000000   ,  \"στS\" -> 0.000000000000   ,  \"στN\" -> 0.000000000000    |>   , \r\"IDS0449_220528_RAW_cal__ref_\" ->   <|    \"ζ\" -> 0.021849716435   ,  \"τ1\" -> 0.033883152649   ,  \"τS\" -> 0.018197027738   ,  \"τN\" -> 0.000213402501   ,  \"τC\" -> 0.001801850307   ,  \"κ0\" -> 0.000000003131   ,  \"mm1\" -> 0.000035185130   ,  \"mm2\" -> 0.020045453610   ,  \"mm3\" -> 0.034417057136   ,  \"T\" -> 0.520000000000   ,  \"B\" -> 6.000000000000   ,  \"θ\" -> 0.000000000000   ,  \"Reoff\" -> 4122448.979591837150   ,  \"Imoff\" -> 0.000000000000   ,  \"στ1\" -> 0.005200135882   ,  \"στS\" -> 0.000196781752   ,  \"στN\" -> 0.000016694885    |>   , \r\"IDS0449_220528_RAW_cal__sam_\" ->   <|    \"ζ\" -> 0.000000000000   ,  \"τ1\" -> 0.000000000000   ,  \"τS\" -> 0.000000000000   ,  \"τN\" -> 0.000000000000   ,  \"τC\" -> 0.000000000000   ,  \"κ0\" -> 0.000000000000   ,  \"mm1\" -> 0.000000000000   ,  \"mm2\" -> 0.000000000000   ,  \"mm3\" -> 0.000000000000   ,  \"T\" -> 0.520000000000   ,  \"B\" -> 6.000000000000   ,  \"θ\" -> 0.000000000000   ,  \"Reoff\" -> 0.000000000000   ,  \"Imoff\" -> 0.000000000000   ,  \"στ1\" -> 0.000000000000   ,  \"στS\" -> 0.000000000000   ,  \"στN\" -> 0.000000000000    |>   , \r\"IDS0450_220528_RAW_cal__ref_\" ->   <|    \"ζ\" -> 0.021729475893   ,  \"τ1\" -> 0.033901786343   ,  \"τS\" -> 0.020153498516   ,  \"τN\" -> 0.000213217921   ,  \"τC\" -> 0.001808973424   ,  \"κ0\" -> 0.000000003806   ,  \"mm1\" -> 0.000035421184   ,  \"mm2\" -> 0.021964202896   ,  \"mm3\" -> 0.034520410198   ,  \"T\" -> 0.620000000000   ,  \"B\" -> 6.000000000000   ,  \"θ\" -> 0.000000000000   ,  \"Reoff\" -> 3061224.489795919510   ,  \"Imoff\" -> 0.000000000000   ,  \"στ1\" -> 0.006296094438   ,  \"στS\" -> 0.000269248074   ,  \"στN\" -> 0.000016264647    |>   , \r\"IDS0450_220528_RAW_cal__sam_\" ->   <|    \"ζ\" -> 0.000000000000   ,  \"τ1\" -> 0.000000000000   ,  \"τS\" -> 0.000000000000   ,  \"τN\" -> 0.000000000000   ,  \"τC\" -> 0.000000000000   ,  \"κ0\" -> 0.000000000000   ,  \"mm1\" -> 0.000000000000   ,  \"mm2\" -> 0.000000000000   ,  \"mm3\" -> 0.000000000000   ,  \"T\" -> 0.620000000000   ,  \"B\" -> 6.000000000000   ,  \"θ\" -> 0.000000000000   ,  \"Reoff\" -> 0.000000000000   ,  \"Imoff\" -> 0.000000000000   ,  \"στ1\" -> 0.000000000000   ,  \"στS\" -> 0.000000000000   ,  \"στN\" -> 0.000000000000    |>   , \r\"IDS0451_220528_RAW_cal__ref_\" ->   <|    \"ζ\" -> 0.019851972634   ,  \"τ1\" -> 0.033846561532   ,  \"τS\" -> 0.023547995636   ,  \"τN\" -> 0.000274131753   ,  \"τC\" -> 0.002984103948   ,  \"κ0\" -> 0.000000005214   ,  \"mm1\" -> 0.000051766319   ,  \"mm2\" -> 0.026018760545   ,  \"mm3\" -> 0.035055182225   ,  \"T\" -> 0.820000000000   ,  \"B\" -> 6.000000000000   ,  \"θ\" -> 0.000000000000   ,  \"Reoff\" -> 40816.326530613005   ,  \"Imoff\" -> 0.000000000000   ,  \"στ1\" -> 0.001908169809   ,  \"στS\" -> 0.000133930876   ,  \"στN\" -> 0.000002638452    |>   , \r\"IDS0451_220528_RAW_cal__sam_\" ->   <|    \"ζ\" -> 0.000000000000   ,  \"τ1\" -> 0.000000000000   ,  \"τS\" -> 0.000000000000   ,  \"τN\" -> 0.000000000000   ,  \"τC\" -> 0.000000000000   ,  \"κ0\" -> 0.000000000000   ,  \"mm1\" -> 0.000000000000   ,  \"mm2\" -> 0.000000000000   ,  \"mm3\" -> 0.000000000000   ,  \"T\" -> 0.820000000000   ,  \"B\" -> 6.000000000000   ,  \"θ\" -> 0.000000000000   ,  \"Reoff\" -> 0.000000000000   ,  \"Imoff\" -> 0.000000000000   ,  \"στ1\" -> 0.000000000000   ,  \"στS\" -> 0.000000000000   ,  \"στN\" -> 0.000000000000    |>   , \r\"IDS0452_220528_RAW_cal__ref_\" ->   <|    \"ζ\" -> 0.016283381951   ,  \"τ1\" -> 0.033904524460   ,  \"τS\" -> 0.031661688913   ,  \"τN\" -> 0.000274537016   ,  \"τC\" -> 0.003250738485   ,  \"κ0\" -> 0.000000007263   ,  \"mm1\" -> 0.000047369067   ,  \"mm2\" -> 0.031583889293   ,  \"mm3\" -> 0.037980260279   ,  \"T\" -> 1.120000000000   ,  \"B\" -> 6.000000000000   ,  \"θ\" -> 0.000000000000   ,  \"Reoff\" -> 40816.326530613005   ,  \"Imoff\" -> 0.000000000000   ,  \"στ1\" -> 0.002257620140   ,  \"στS\" -> 0.000162839807   ,  \"στN\" -> 0.000009699550    |>   , \r\"IDS0452_220528_RAW_cal__sam_\" ->   <|    \"ζ\" -> 0.000000000000   ,  \"τ1\" -> 0.000000000000   ,  \"τS\" -> 0.000000000000   ,  \"τN\" -> 0.000000000000   ,  \"τC\" -> 0.000000000000   ,  \"κ0\" -> 0.000000000000   ,  \"mm1\" -> 0.000000000000   ,  \"mm2\" -> 0.000000000000   ,  \"mm3\" -> 0.000000000000   ,  \"T\" -> 1.120000000000   ,  \"B\" -> 6.000000000000   ,  \"θ\" -> 0.000000000000   ,  \"Reoff\" -> 0.000000000000   ,  \"Imoff\" -> 0.000000000000   ,  \"στ1\" -> 0.000000000000   ,  \"στS\" -> 0.000000000000   ,  \"στN\" -> 0.000000000000    |>   , \r\"IDS0453_220529_RAW_cal__ref_\" ->   <|    \"ζ\" -> 0.018860897000   ,  \"τ1\" -> 0.033783692310   ,  \"τS\" -> 0.033495916545   ,  \"τN\" -> 0.000426157498   ,  \"τC\" -> 0.003160296043   ,  \"κ0\" -> 0.000000011406   ,  \"mm1\" -> 0.000053621310   ,  \"mm2\" -> 0.031431982647   ,  \"mm3\" -> 0.040020259184   ,  \"T\" -> 1.700000000000   ,  \"B\" -> 6.000000000000   ,  \"θ\" -> 0.000000000000   ,  \"Reoff\" -> -371428.571428571827   ,  \"Imoff\" -> 0.000000000000   ,  \"στ1\" -> 0.008605835969   ,  \"στS\" -> 0.000457782614   ,  \"στN\" -> 0.000070271904    |>   , \r\"IDS0453_220529_RAW_cal__sam_\" ->   <|    \"ζ\" -> 0.000000000000   ,  \"τ1\" -> 0.000000000000   ,  \"τS\" -> 0.000000000000   ,  \"τN\" -> 0.000000000000   ,  \"τC\" -> 0.000000000000   ,  \"κ0\" -> 0.000000000000   ,  \"mm1\" -> 0.000000000000   ,  \"mm2\" -> 0.000000000000   ,  \"mm3\" -> 0.000000000000   ,  \"T\" -> 1.700000000000   ,  \"B\" -> 6.000000000000   ,  \"θ\" -> 0.000000000000   ,  \"Reoff\" -> 0.000000000000   ,  \"Imoff\" -> 0.000000000000   ,  \"στ1\" -> 0.000000000000   ,  \"στS\" -> 0.000000000000   ,  \"στN\" -> 0.000000000000    |>   , \r\"IDS0454_220529_RAW_cal__ref_\" ->   <|    \"ζ\" -> 0.017534515106   ,  \"τ1\" -> 0.023238617838   ,  \"τS\" -> 0.014265591932   ,  \"τN\" -> 0.000383027801   ,  \"τC\" -> 0.002949269667   ,  
